vi "Create Random Maze.vi"(8 "error in (no error)":errorcluster, 9 "Height (40)":i32=40, 10 "Width (40)":i32=40, 11 "Maze Level":T1) -> (0 "error out":errorcluster, 3 "Maze":refnum<class "Maze.lvclass">)   [LabVIEW 2020, in "Maze.lvlib" / "MazeGen.lvclass"]
doc: "Creates a maze of the specified level. Except for the <b>Basic</b> level all higher level generators are loaded dynamically from disk so they can be distributed individually after the challenge begins.\n\n<b>Errors</b>\n\n<b>-124100</b> is thrown if the PPL/class of the generator for the specified level is unable to be loaded."
uses:
  MazeGen.lvclass
  Maze Level.ctl
  Maze/Maze.lvclass
  Maze.lvlib
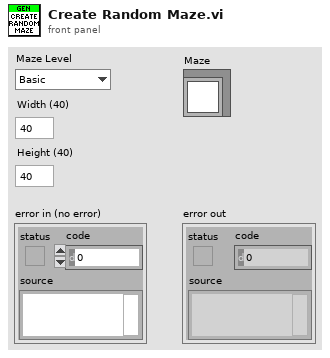
[diagram p1: front panel]
types:
  T1 = typedef "Maze.lvlib/Maze Level.ctl" = enum16{"Basic", "Intermediate", "Advanced", "Quantum"}
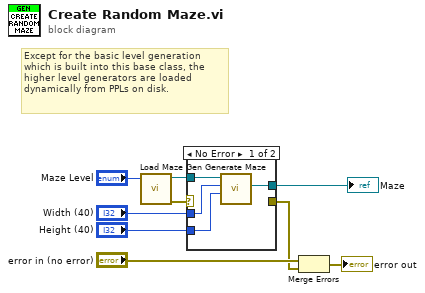
[diagram p0: block diagram]
diagram:
  # "Except for the basic level generation which is built into this base class, the higher level generators are loaded dynamically from PPLs on disk."
  n1 = call "Load Maze Gen.vi"("Maze Level"="Maze Level") -> ("error out"=w7:errorcluster, "MazeGen"=w6:refnum<class "MazeGen.lvclass">)  [unwired: 9 in]
  n2 = case shown="No Error" w7 {
    selector: w7 -> [_ w14]
    tunnel: w6 -> [w13 _]
    tunnel: "Width (40)" -> [w12 _]
    tunnel: "Height (40)" -> [w11 _]
    tunnel: [w10 _] -> w3
    tunnel: [_ w14] -> w1
    frame No Error {
      n3 = call-dynamic "Generate Maze.vi"("Height"=w11, "Width"=w12, "MazeGen in"=w13) -> ("Maze"=w10:refnum<class "Maze.lvclass">)  [unwired: 6 in, 2 out]
    }
    frame Error {
    }
  }
  "Maze" <- w3
  n4 = Merge Errors("error in (no error)", w1) -> (→"error out":errorcluster)
